vi "HIL Setup.vi"() -> ()   [LabVIEW 2012]
uses:
  Page.ctl
panel:
  out "Numeric 3":i32
  out "Numeric 2":i32
  out "Numeric":i32
  in  "Cancel Button":bool
  in  "Next Button":bool
  in  "Tab Control":T1(tab)
  in  "num1":u16
  in  "num2":u16
  in  "num3":u16
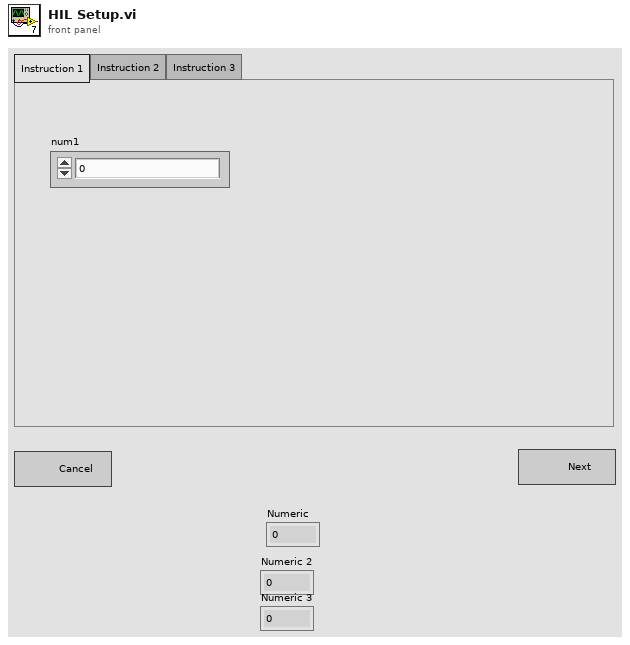
[diagram p1: front panel]
types:
  T1 = enum32{"Instruction 1", "Instruction 2", "Instruction 3"}
  T2 = typedef "Page.ctl" = enum16{"1", "2", "3"}
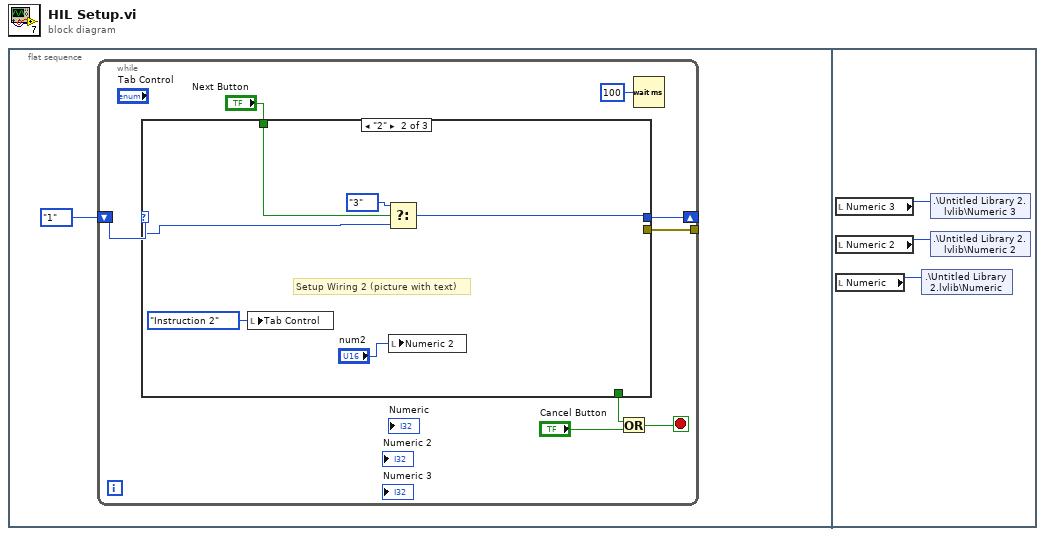
[diagram p0: block diagram]
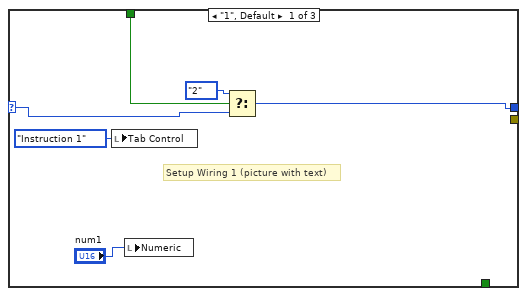
[diagram p2: hidden frame]
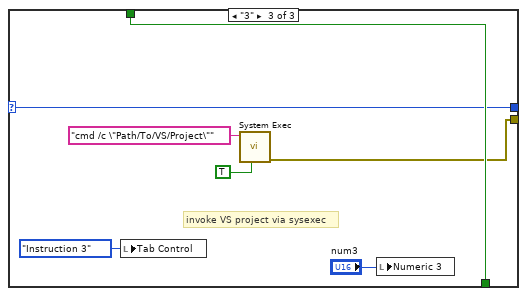
[diagram p3: hidden frame]
diagram:
  n1 = flat-sequence {
    frame #0 {
      n2 = while {
        shift-right: [w8] -> _
        shift-left: Page."1" ("Page") -> [w9]
        tunnel: [w2] -> _
        stop <- w6 stop-if-true
        n3 = case shown="\"2\"" w9 {
          selector: w9 -> [w10 w19 w25]
          tunnel: [w15 w18 w25] -> w8
          tunnel: "Next Button" -> [w13 w20 w28]
          tunnel: [_ _ w28] -> w4
          tunnel: [_ _ w24] -> w2
          frame "1", Default {
            # "Setup Wiring 1 (picture with text)"
            n4 = local write "Tab Control"(T1."Instruction 1" ("Tab Control")) -> ()
            n5 = local write "Numeric"("num1") -> ()
            n6 = Select(t=Page."2" ("Page"), s=w13, f=w10) -> (s? t:f=w15:T2)
          }
          frame "2" {
            # "Setup Wiring 2 (picture with text)"
            n7 = local write "Tab Control"(T1."Instruction 2" ("Tab Control")) -> ()
            n8 = Select(t=Page."3" ("Page"), s=w20, f=w19) -> (s? t:f=w18:T2)
            n9 = local write "Numeric 2"("num2") -> ()
          }
          frame "3" {
            # "invoke VS project via sysexec"
            n10 = local write "Tab Control"(T1."Instruction 3" ("Tab Control")) -> ()
            n11 = call <vilib>:"System Exec.vi"("run minimized? (F)"=TRUE, "command line"="cmd /c \"Path/To/VS/Project\"") -> ("error out"=w24:errorcluster)  [unwired: 6 in, 3 out]
            n12 = local write "Numeric 3"("num3") -> ()
          }
        }
        n13 = Or(x=w4, y="Cancel Button") -> (x .or. y?=w6:bool)
        n14 = Wait (ms)(milliseconds to wait=u32 100) -> ()  [unwired: 1 out]
      }
    }
    frame #1 {
      n15 = local read "Numeric 3"() -> (w29:i32)
      n16 = local read "Numeric 2"() -> (w30:i32)
      n17 = local read "Numeric"() -> (w31:i32)
      n18 = shared-variable ".\\Untitled Library 2.lvlib\\Numeric"(w31) -> ()  [unwired: 1 in, 1 out]
      n19 = shared-variable ".\\Untitled Library 2.lvlib\\Numeric 3"(w29) -> ()  [unwired: 1 in, 1 out]
      n20 = shared-variable ".\\Untitled Library 2.lvlib\\Numeric 2"(w30) -> ()  [unwired: 1 in, 1 out]
    }
  }
